vi "Global Sensor Reads.vi"() -> ()   [LabVIEW 2020]
panel:
  in  "Target Locked?":bool
  in  "Distance to Target (in)":dbl
  in  "Limelight Connected":bool
  in  "Target Acquired?":bool
  in  "Camera Goal (Y) (deg)":dbl
  in  "Camera Goal (X) (deg)":dbl
  in  "Robot Left Side Position":dbl
  in  "Robot Right Side Position":dbl
  in  "Climber out?":bool
  in  "Intake out?":bool
  in  "Accelerator Speed":dbl
  in  "Indexer Speed":dbl
  in  "Robot Left Side Speed":dbl
  in  "Robot Right Side Speed":dbl
  in  "Shooter Speed":dbl
  in  "Robot Angular Velocity":dbl
  in  "Robot Angle":dbl
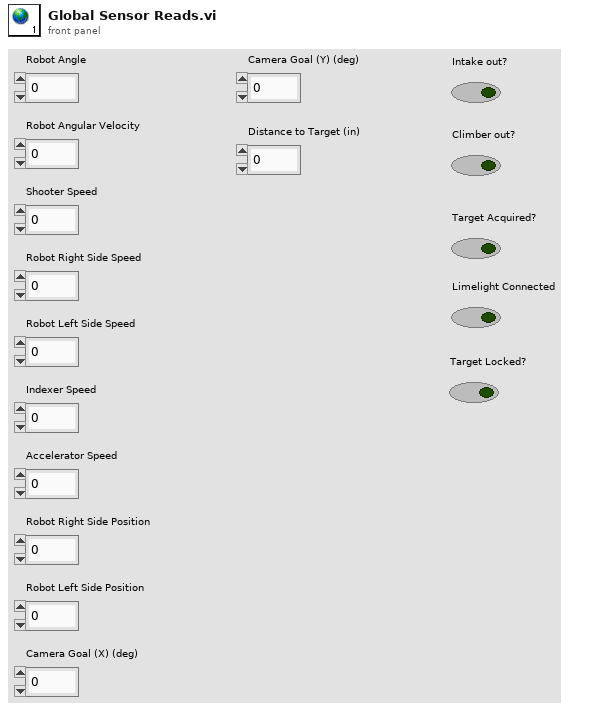
[diagram p1: front panel]
diagram:
